vi "Test External TCP.vi"() -> ()   [LabVIEW 2020]
uses:
  lv-http-util/HTTP Utils/Request/Request.lvclass
  lv-http-util/HTTP Utils/Response/Response.lvclass
  Stream-Websocket/Websocket Server/Websocket Server.lvclass
  lv-stream/stream/Stream/Stream.lvclass
  Stream-Websocket/Stream-Websocket.lvlib
  lv-stream/stream/URI/URI.lvclass
  Stream-Websocket/Websocket Client/Websocket Client.lvclass
  Stream-Websocket/WebSocketUpgradeResponse/WebSocketUpgradeResponse.lvclass
panel:
  in  "WS Port":u16=4663
  out "HTTP":errorcluster
  in  "HTTP Port":u16=7080
  out "WS":errorcluster
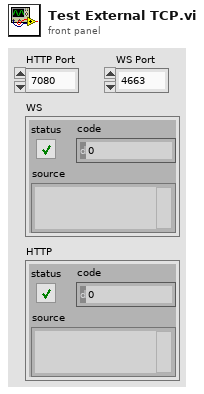
[diagram p1: front panel]
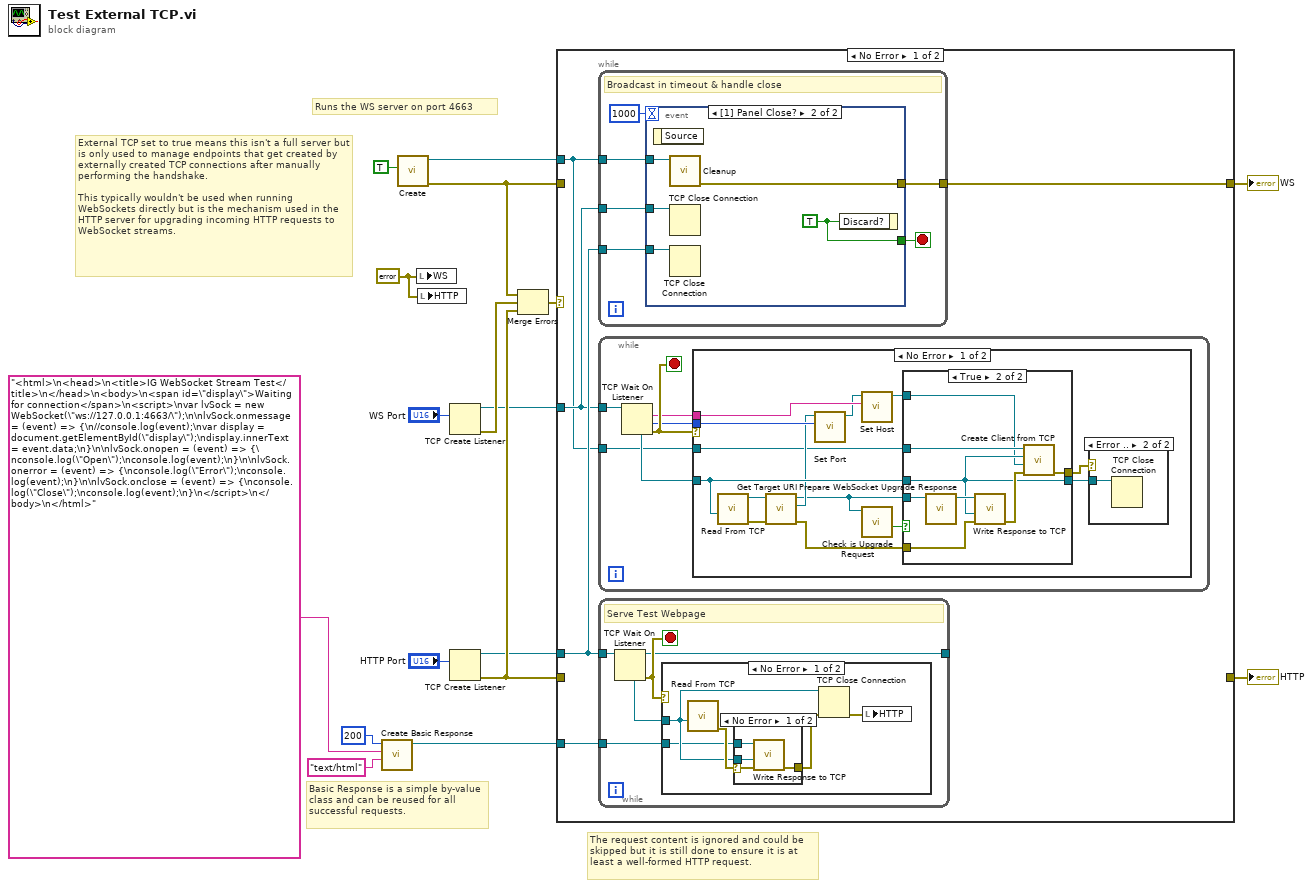
[diagram p0: block diagram]
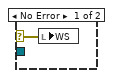
[diagram p2: hidden frame]
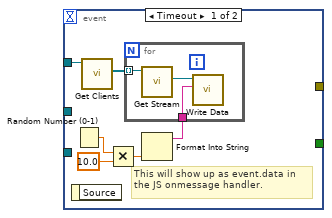
[diagram p5: hidden frame]
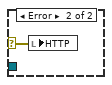
[diagram p7: hidden frame]
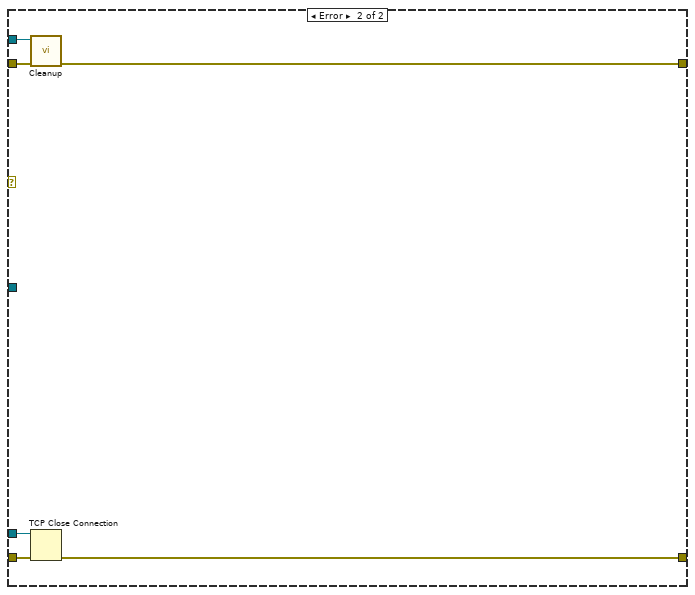
[diagram p8: hidden frame]
diagram:
  w11 = errorcluster {"status"=FALSE, "code"=0, "source"=""} ("WS")
  # "External TCP set to true means this isn't a full server but is only used to manage endpoints that get created by externally created TCP connections after manually performing the handshake.\n\nThis typically wouldn't be used when running WebSockets directly but is the mechanism used in the HTTP server for upgrading incoming HTTP requests to WebSocket streams."
  # "The request content is ignored and could be skipped but it is still done to ensure it is at least a well-formed HTTP request."
  # "Basic Response is a simple by-value class and can be reused for all successful requests."
  # "Runs the WS server on port 4663"
  n1 = call "Create Basic Response.vi"("Content-Type (text/plain)"="text/html", "Payload"="<html>\n<head>\n<title>IG WebSocket Stream Test</title>\n</head>\n<body>\n<span id=\"display\">Waiting for connection</span>\n<script>\nvar lvSock = new WebSocket(\"ws://127.0.0.1:4663/\");\n\nlvSock.onmessage = (event) => {\n//console.log(event);\nvar display = document.getElementById(\"display\");\ndisplay.innerText = event.data;\n}\n\nlvSock.onopen = (event) => {\nconsole.log(\"Open\");\nconsole.log(event);\n}\n\nlvSock.onerror = (event) => {\nconsole.log(\"Error\");\nconsole.log(event);\n}\n\nlvSock.onclose = (event) => {\nconsole.log(\"Close\");\nconsole.log(event);\n}\n</script>\n</body>\n</html>", "Status Code"=u16 200) -> ("Response out"=w13:refnum<class "Response.lvclass">)  [unwired: 7 in, 1 out]
  n2 = call "Create.vi"("External TCP? (False)"=TRUE ("Callbacks Only? (False)")) -> ("error out"=w1:errorcluster, "Websocket Server out"=w2:refnum<class "Websocket Server.lvclass">)  [unwired: 9 in]
  n3 = local write "WS"(w11) -> ()
  n4 = local write "HTTP"(w11) -> ()
  n5 = TCP Create Listener(10:"WS Port") -> (0:w16:errorcluster, 3:w3:refnum<k5>)  [unwired: 4 in, 1 out]
  n6 = TCP Create Listener(10:"HTTP Port") -> (0:w17:errorcluster, 3:w9:refnum<k5>)  [unwired: 4 in, 1 out]
  n7 = Merge Errors(w1, w16, w17) -> (w8:errorcluster)
  n8 = case shown="No Error" w8 {
    tunnel: w13 -> [w22 _]
    tunnel: w2 -> [w18 w95]
    tunnel: w9 -> [w21 w93]
    tunnel: w1 -> [_ w96]
    tunnel: w17 -> [_ w92]
    tunnel: [_ w91] -> w7
    tunnel: [w20 w94] -> w6
    tunnel: w3 -> [w19 _]
    frame No Error {
      n9 = while {
        tunnel: w21 -> [w60]
        tunnel: w18 -> [w58]
        tunnel: [w56] -> w20
        tunnel: w19 -> [w55]
        stop <- w59 stop-if-true
        # "Broadcast in timeout & handle close"
        n10 = event shown="[1] Panel Close?" {
          selector: _ -> [_ _]
          dyn-events: _ -> [_ _]
          timeout: 1000 -> [_ _]
          tunnel: w60 -> [_ w74]
          tunnel: [_ w73] -> w59
          tunnel: w58 -> [w66 w72]
          tunnel: [_ w71] -> w56
          tunnel: w55 -> [_ w70]
          event Timeout {
            # "This will show up as event.data in the JS onmessage handler."
            n11 = event-data() -> ()  [unwired: 1 in, 1 out]
            n12 = Random Number (0-1)() -> (number: 0 to 1=w65:dbl)
            n13 = call "Get Clients.vi"("Websocket Server in"=w66) -> ("Clients"=w62:refnum<class "Websocket Client.lvclass">[])  [unwired: 8 in, 2 out]
            n14 = Multiply(x=w65, y=10.0) -> (x*y=w63:dbl)
            n15 = Format Into String(w63) -> (resulting string=w61:string)  [unwired: 3 in, 1 out]
            n16 = for {
              tunnel: w62 -> [w68] mode=indexing
              tunnel: w61 -> [w69]
              n17 = call-dynamic "Get Stream.vi"("Websocket Client in"=w68) -> ("Stream"=w67:refnum<class "Stream.lvclass">)  [unwired: 8 in, 2 out]
              n18 = call "Write Data.vi"("Data"=w69, "Stream in"=w67) -> ()  [unwired: 8 in, 2 out]
            }
          }
          event Panel Close? {
            w73 = TRUE ("Discard?")
            n19 = event-data() -> ()  [unwired: 1 in, 1 out]
            n20 = call-dynamic "Cleanup.vi"("Websocket Server in"=w72) -> ("error out"=w71:errorcluster)  [unwired: 10 in]
            n21 = TCP Close Connection(connection ID=w70) -> ()  [unwired: 2 in, 2 out]
            n22 = TCP Close Connection(connection ID=w74) -> ()  [unwired: 2 in, 2 out]
            n23 = event-data("Discard?"=w73) -> ()  [unwired: 1 in, 1 out]
          }
        }
      }
      n24 = while {
        tunnel: w19 -> [w28]
        tunnel: w18 -> [w23]
        stop <- w26 stop-if-true
        n25 = TCP Wait On Listener(11:w28) -> (0:w26:errorcluster, 1:w24:u16, 2:w25:string, 4:w27:refnum<k5>)  [unwired: 3 in, 1 out]
        n26 = case shown="No Error" w26 {
          tunnel: w27 -> [w41 _]
          tunnel: w25 -> [w39 _]
          tunnel: w24 -> [w37 _]
          tunnel: w23 -> [w32 _]
          frame No Error {
            n27 = call "Read From TCP.vi"("TCP Connection"=w41) -> ("error out"=w31:errorcluster, "Request out"=w40:refnum<class "Request.lvclass">)  [unwired: 9 in]
            n28 = call "Get Target URI.vi"("error in (no error)"=w31, "Request in"=w40) -> ("error out"=w42:errorcluster, "Target URI"=w36:refnum<class "URI.lvclass">, "Request out"=w33:refnum<class "Request.lvclass">)  [unwired: 7 in]
            n29 = call "Set Port.vi"("Port"=w37, "URI in"=w36) -> ("URI out"=w38:refnum<class "URI.lvclass">)  [unwired: 8 in, 1 out]
            n30 = call "Set Host.vi"("Host"=w39, "URI in"=w38) -> ("URI out"=w34:refnum<class "URI.lvclass">)  [unwired: 8 in, 1 out]
            n31 = call "Check is Upgrade Request.vi"("Request in"=w33) -> ("Upgrade Request?"=w35:bool)  [unwired: 7 in, 3 out]
            n32 = case shown="True" w35 {
              tunnel: w41 -> [w45 w49]
              tunnel: w34 -> [_ w48]
              tunnel: w33 -> [_ w54]
              tunnel: w32 -> [_ w53]
              tunnel: [w45 w49] -> w29
              tunnel: w42 -> [w46 w50]
              tunnel: [w46 w47] -> w30
              frame False {
              }
              frame True {
                n33 = call "Prepare WebSocket Upgrade Response.vi"("Request"=w54) -> ("WebSocket Response"=w52:refnum<class "WebSocketUpgradeResponse.lvclass">)  [unwired: 10 in]
                n34 = call "Write Response to TCP.vi"("error in (no error)"=w50, "TCP Connection"=w49, "Response in"=w52) -> ("error out"=w51:errorcluster)  [unwired: 7 in, 1 out]
                n35 = call "Create Client from TCP.vi"("error in (no error)"=w51, "URI"=w48, "TCP Connection"=w49, "Websocket Server in"=w53) -> ("error out"=w47:errorcluster)  [unwired: 6 in, 1 out]
              }
            }
            n36 = case shown="Error .." w30 {
              selector: w30 -> [w43 _]
              tunnel: w29 -> [_ w44]
              frame No Error {
                n37 = local write "WS"(w43) -> ()
              }
              frame Error {
                n38 = TCP Close Connection(connection ID=w44) -> ()  [unwired: 2 in, 2 out]
              }
            }
          }
          frame Error {
          }
        }
      }
      n39 = while {
        tunnel: w21 -> [w79]
        tunnel: w22 -> [w76]
        tunnel: [w75] -> _
        stop <- w78 stop-if-true
        # "Serve Test Webpage"
        n40 = TCP Wait On Listener(11:w79) -> (0:w78:errorcluster, 3:w75:refnum<k5>, 4:w77:refnum<k5>)  [unwired: 3 in, 2 out]
        n41 = case shown="No Error" w78 {
          selector: w78 -> [_ w90]
          tunnel: w77 -> [w83 _]
          tunnel: w76 -> [w81 _]
          frame No Error {
            n42 = call "Read From TCP.vi"("TCP Connection"=w83) -> ("error out"=w84:errorcluster)  [unwired: 9 in, 1 out]
            n43 = case shown="No Error" w84 {
              selector: w84 -> [w88 w89]
              tunnel: w81 -> [w87 _]
              tunnel: w83 -> [w86 _]
              tunnel: [w85 w89] -> w82
              frame No Error {
                n44 = call "Write Response to TCP.vi"("error in (no error)"=w88, "TCP Connection"=w86, "Response in"=w87) -> ("error out"=w85:errorcluster)  [unwired: 7 in, 1 out]
              }
              frame Error {
              }
            }
            n45 = TCP Close Connection(connection ID=w83, error in (no error)=w82) -> (error out=w80:errorcluster)  [unwired: 1 in, 1 out]
            n46 = local write "HTTP"(w80) -> ()
          }
          frame Error {
            n47 = local write "HTTP"(w90) -> ()
          }
        }
      }
    }
    frame Error {
      n48 = call-dynamic "Cleanup.vi"("error in (no error)"=w96, "Websocket Server in"=w95) -> ("error out"=w94:errorcluster)  [unwired: 9 in]
      n49 = TCP Close Connection(connection ID=w93, error in (no error)=w92) -> (error out=w91:errorcluster)  [unwired: 1 in, 1 out]
    }
  }
  "WS" <- w6
  "HTTP" <- w7
